vi "local+global.vi"() -> ()   [LabVIEW 2015]
uses:
  Global 1.vi
panel:
  out "Numeric":dbl
  out "String":string
  in  "abr":string
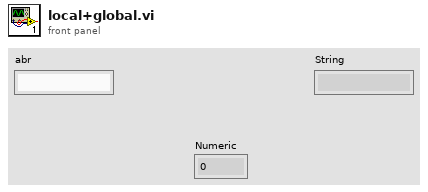
[diagram p1: front panel]
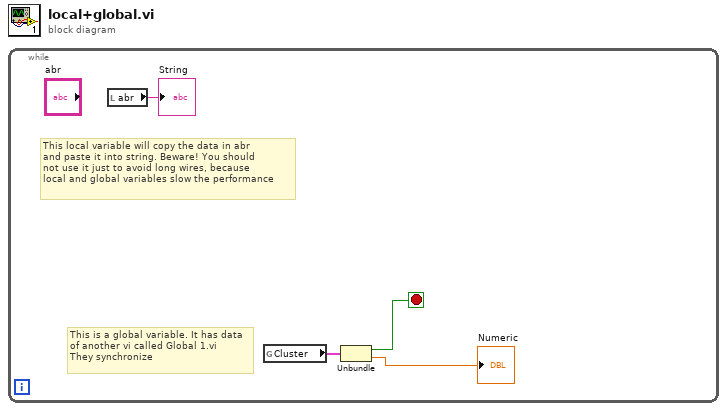
[diagram p0: block diagram]
diagram:
  n1 = while {
    stop <- w2 stop-if-true
    # "This is a global variable. It has data\nof another vi called Global 1.vi\nThey synchronize"
    # "This local variable will copy the data in abr \nand paste it into string. Beware! You should\nnot use it just to avoid long wires, because\nlocal and global variables slow the performance"
    n2 = local read "abr"() -> (→"String":string)
    n3 = global read "Global 1.vi" "Cluster"() -> (w3:cluster{"bol1":bool, "Num1":dbl})
    n4 = Unbundle(w3) -> ("bol1"=w2:bool, "Num1"=→"Numeric":dbl)
  }
